vi "Read FPGA Session.vi"(8 "error in (no error)":errorcluster, 11 "gController in":refnum<class "gController.lvclass">) -> (0 "error out":errorcluster, 2 "FPGA Session":refnum<data-value>, 3 "gController out":refnum<class "gController.lvclass">)   [LabVIEW 2017, in "Controller.lvlib" / "gController.lvclass"]
uses:
  gController.lvclass
  Session/Raw FPGA/FPGA Session.lvclass
  gController.lvclass/gController.ctl
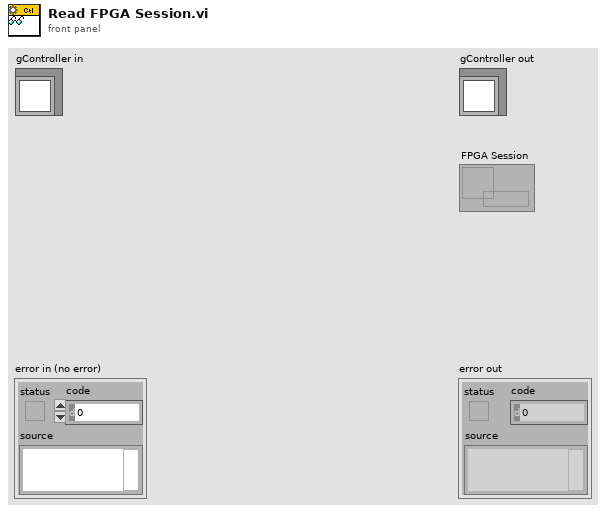
[diagram p1: front panel]
types:
  T1 = typedef "Session - Root.lvclass/Session Handle.ctl" = refnum<data-value>
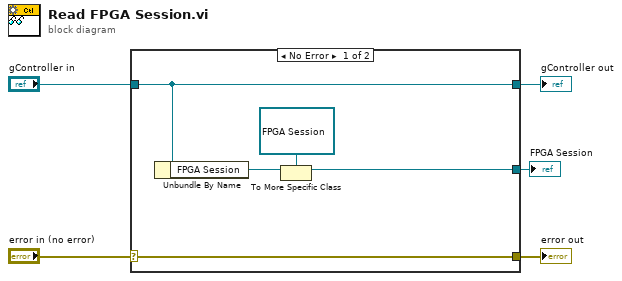
[diagram p0: block diagram]
diagram:
  n1 = case shown="No Error" "error in (no error)" {
    selector: "error in (no error)" -> [w10 w11]
    tunnel: [w10 w11] -> w4
    tunnel: [w9 w12] -> w2
    tunnel: "gController in" -> [w9 w12]
    tunnel: [w6 _] -> w1
    frame No Error {
      n2 = Unbundle By Name(w9) -> ("FPGA Session"=w8:T1)
      n3 = To More Specific Class(target class=refnum<data-value> refnum, reference=w8) -> (specific class reference=w6:refnum<data-value>)  [unwired: 1 in, 1 out]
    }
    frame Error {
    }
  }
  "error out" <- w4
  "gController out" <- w2
  "FPGA Session" <- w1
